vi "Link Control References.vi"(8 "error in (no error)":errorcluster, 10 "Control References":T1[](array[typedef]), 11 "Main in":refnum<class "Main.lvclass">) -> (0 "error out":errorcluster, 3 "Main out":refnum<class "Main.lvclass">)   [LabVIEW 2023, in "Main.lvlib" / "Main.lvclass"]
doc: "<b> Link Control References </b>\n<b> Engine Level </b>\nThis is the base abstraction layer. The purpose of this method is to link the control references to the class private data."
uses:
  Library/Main.lvclass
  builds/Framework/Engine.lvlibp/Engine/Custom Controls/Control Reference.ctl
  Library/Main.lvclass/Main.ctl
  builds/Framework/Engine.lvlibp/Engine/Accessors/Read Version.vi
  builds/Framework/Panel Manager.lvlibp/Panel/Panel/Subpanel/Subpanel.vi
  builds/Framework/Panel Manager.lvlibp/Panel/Panel.lvlib
  builds/Framework/Panel Manager.lvlibp/Panel/Panel/Subpanel/Subpanel.lvclass
  builds/Framework/Engine.lvlibp/Engine/Library/Engine.lvclass
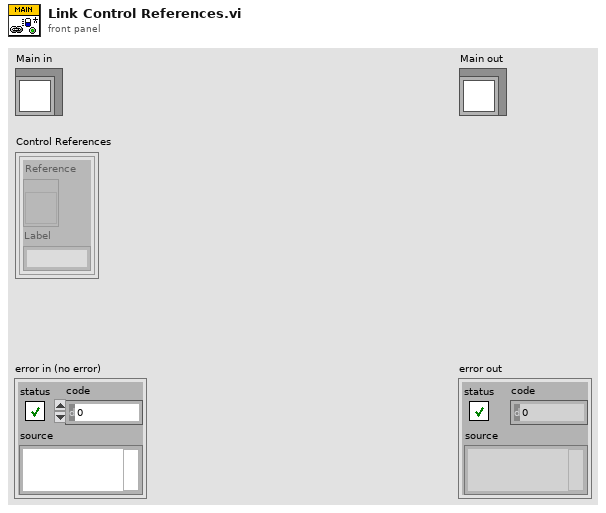
[diagram p1: front panel]
types:
  T1 = typedef "Engine.lvlibp/Engine.lvclass/Control Reference.ctl" = cluster{"Reference":refnum<vi>, "Label":string}
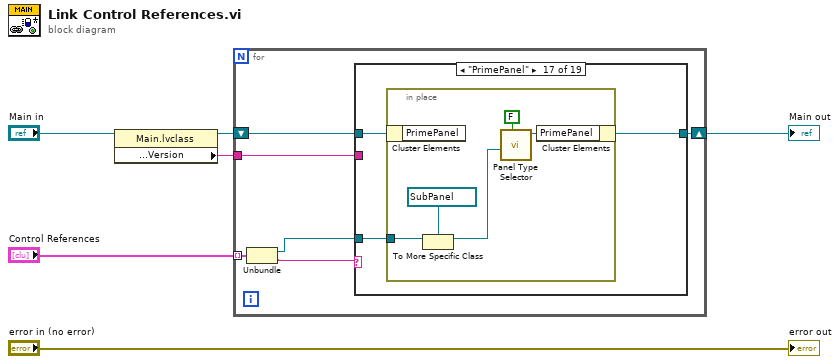
[diagram p0: block diagram]
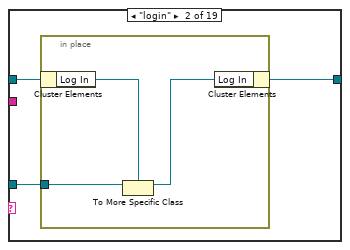
[diagram p3: hidden frame]
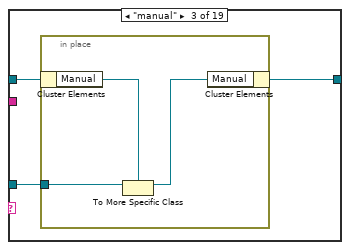
[diagram p4: hidden frame]
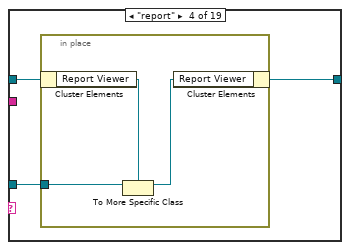
[diagram p5: hidden frame]
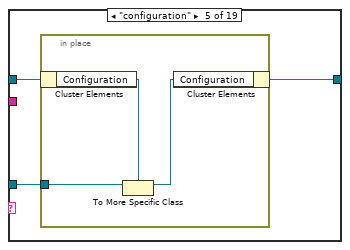
[diagram p6: hidden frame]
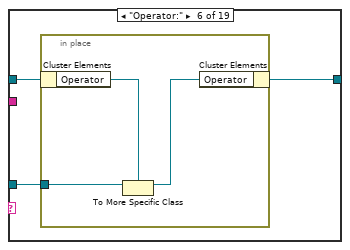
[diagram p7: hidden frame]
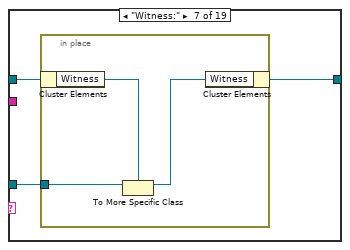
[diagram p8: hidden frame]
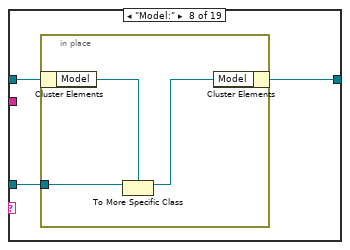
[diagram p9: hidden frame]
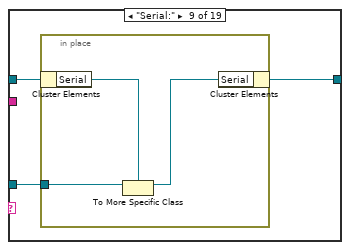
[diagram p10: hidden frame]
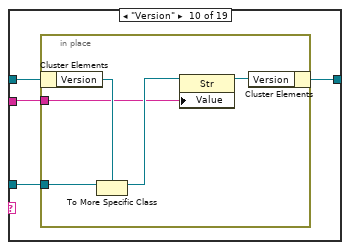
[diagram p11: hidden frame]
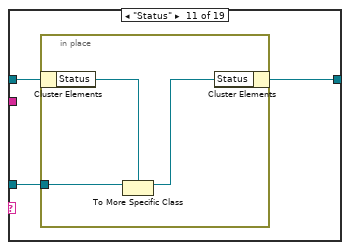
[diagram p12: hidden frame]
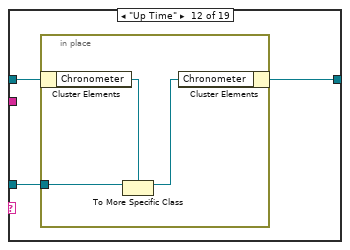
[diagram p13: hidden frame]
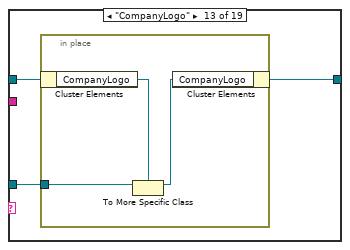
[diagram p14: hidden frame]
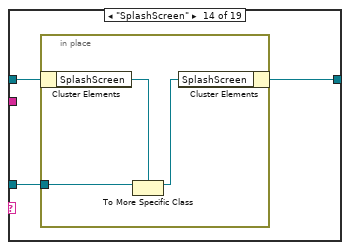
[diagram p15: hidden frame]
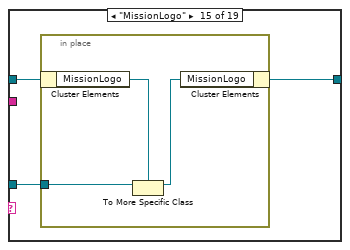
[diagram p16: hidden frame]
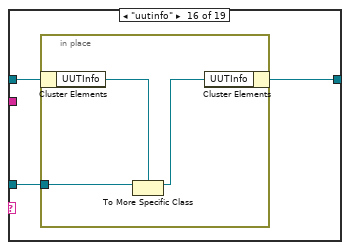
[diagram p17: hidden frame]
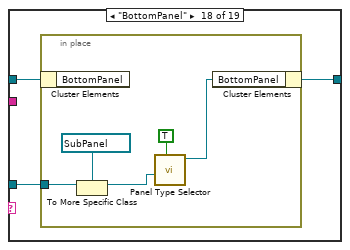
[diagram p18: hidden frame]
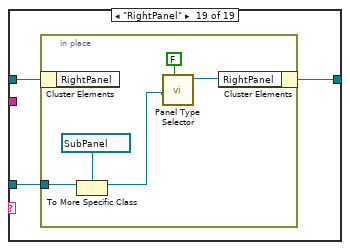
[diagram p19: hidden frame]
diagram:
  n1 = property class="Main.lvclass"(reference="Main in") -> (reference out=w2:refnum<class "Main.lvclass">, "Accessors:Configuration:Version"=w1:string)  [unwired: 1 in, 1 out]
  n2 = for {
    shift-right: [w11] -> w3
    shift-left: w2 -> [w12]
    tunnel: w1 -> [w10]
    tunnel: "Control References" -> [w9] mode=indexing
    n3 = Unbundle(w9) -> ("Reference"=w7:refnum<vi>, "Label"=w8:string)
    n4 = case shown="\"PrimePanel\"" w8 {
      tunnel: w7 -> [_ w14 w20 w26 w32 w38 w44 w50 w56 w63 w71 w77 w83 w89 w95 w101 w107 w115 w123]
      tunnel: w12 -> [w13 w16 w22 w28 w34 w40 w46 w52 w58 w65 w73 w79 w85 w91 w97 w103 w109 w117 w125]
      tunnel: [w13 w15 w21 w27 w33 w39 w45 w51 w57 w64 w72 w78 w84 w90 w96 w102 w108 w116 w124] -> w11
      tunnel: w10 -> [_ _ _ _ _ _ _ _ _ w62 _ _ _ _ _ _ _ _ _]
      frame "False", Default {
      }
      frame "login" {
        n5 = in-place {
          in-place-border: w14 -> [w18]
          n6 = in-place-cluster #1(w16) -> ("Log In"=w19:refnum<vi>)
          n7 = To More Specific Class(target class=w19, reference=w18) -> (specific class reference=w17:refnum<vi>)  [unwired: 1 in, 1 out]
          n8 = in-place-cluster #1("Log In"=w17) -> (w15:refnum<class "Main.lvclass">)
        }
      }
      frame "manual" {
        n9 = in-place {
          in-place-border: w20 -> [w24]
          n10 = in-place-cluster #2(w22) -> ("Manual"=w25:refnum<vi>)
          n11 = To More Specific Class(target class=w25, reference=w24) -> (specific class reference=w23:refnum<vi>)  [unwired: 1 in, 1 out]
          n12 = in-place-cluster #2("Manual"=w23) -> (w21:refnum<class "Main.lvclass">)
        }
      }
      frame "report" {
        n13 = in-place {
          in-place-border: w26 -> [w30]
          n14 = in-place-cluster #3(w28) -> ("Report Viewer"=w31:refnum<vi>)
          n15 = To More Specific Class(target class=w31, reference=w30) -> (specific class reference=w29:refnum<vi>)  [unwired: 1 in, 1 out]
          n16 = in-place-cluster #3("Report Viewer"=w29) -> (w27:refnum<class "Main.lvclass">)
        }
      }
      frame "configuration" {
        n17 = in-place {
          in-place-border: w32 -> [w36]
          n18 = in-place-cluster #4(w34) -> ("Configuration"=w37:refnum<vi>)
          n19 = To More Specific Class(target class=w37, reference=w36) -> (specific class reference=w35:refnum<vi>)  [unwired: 1 in, 1 out]
          n20 = in-place-cluster #4("Configuration"=w35) -> (w33:refnum<class "Main.lvclass">)
        }
      }
      frame "Operator:" {
        n21 = in-place {
          in-place-border: w38 -> [w42]
          n22 = in-place-cluster #5(w40) -> ("Operator"=w43:refnum<vi>)
          n23 = To More Specific Class(target class=w43, reference=w42) -> (specific class reference=w41:refnum<vi>)  [unwired: 1 in, 1 out]
          n24 = in-place-cluster #5("Operator"=w41) -> (w39:refnum<class "Main.lvclass">)
        }
      }
      frame "Witness:" {
        n25 = in-place {
          in-place-border: w44 -> [w48]
          n26 = in-place-cluster #6(w46) -> ("Witness"=w49:refnum<vi>)
          n27 = To More Specific Class(target class=w49, reference=w48) -> (specific class reference=w47:refnum<vi>)  [unwired: 1 in, 1 out]
          n28 = in-place-cluster #6("Witness"=w47) -> (w45:refnum<class "Main.lvclass">)
        }
      }
      frame "Model:" {
        n29 = in-place {
          in-place-border: w50 -> [w54]
          n30 = in-place-cluster #7(w52) -> ("Model"=w55:refnum<vi>)
          n31 = To More Specific Class(target class=w55, reference=w54) -> (specific class reference=w53:refnum<vi>)  [unwired: 1 in, 1 out]
          n32 = in-place-cluster #7("Model"=w53) -> (w51:refnum<class "Main.lvclass">)
        }
      }
      frame "Serial:" {
        n33 = in-place {
          in-place-border: w56 -> [w60]
          n34 = in-place-cluster #8(w58) -> ("Serial"=w61:refnum<vi>)
          n35 = To More Specific Class(target class=w61, reference=w60) -> (specific class reference=w59:refnum<vi>)  [unwired: 1 in, 1 out]
          n36 = in-place-cluster #8("Serial"=w59) -> (w57:refnum<class "Main.lvclass">)
        }
      }
      frame "Version" {
        n37 = in-place {
          in-place-border: w63 -> [w69]
          in-place-border: w62 -> [w66]
          n38 = in-place-cluster #9(w65) -> ("Version"=w70:refnum<vi>)
          n39 = To More Specific Class(target class=w70, reference=w69) -> (specific class reference=w68:refnum<vi>)  [unwired: 1 in, 1 out]
          n40 = property class="Str"(reference=w68, "Value"=w66) -> (reference out=w67:refnum<vi>)  [unwired: 1 in, 1 out]
          n41 = in-place-cluster #9("Version"=w67) -> (w64:refnum<class "Main.lvclass">)
        }
      }
      frame "Status" {
        n42 = in-place {
          in-place-border: w71 -> [w75]
          n43 = in-place-cluster #10(w73) -> ("Status"=w76:refnum<vi>)
          n44 = To More Specific Class(target class=w76, reference=w75) -> (specific class reference=w74:refnum<vi>)  [unwired: 1 in, 1 out]
          n45 = in-place-cluster #10("Status"=w74) -> (w72:refnum<class "Main.lvclass">)
        }
      }
      frame "Up Time" {
        n46 = in-place {
          in-place-border: w77 -> [w81]
          n47 = in-place-cluster #11(w79) -> ("Chronometer"=w82:refnum<vi>)
          n48 = To More Specific Class(target class=w82, reference=w81) -> (specific class reference=w80:refnum<vi>)  [unwired: 1 in, 1 out]
          n49 = in-place-cluster #11("Chronometer"=w80) -> (w78:refnum<class "Main.lvclass">)
        }
      }
      frame "CompanyLogo" {
        n50 = in-place {
          in-place-border: w83 -> [w87]
          n51 = in-place-cluster #12(w85) -> ("CompanyLogo"=w88:refnum<vi>)
          n52 = To More Specific Class(target class=w88, reference=w87) -> (specific class reference=w86:refnum<vi>)  [unwired: 1 in, 1 out]
          n53 = in-place-cluster #12("CompanyLogo"=w86) -> (w84:refnum<class "Main.lvclass">)
        }
      }
      frame "SplashScreen" {
        n54 = in-place {
          in-place-border: w89 -> [w93]
          n55 = in-place-cluster #13(w91) -> ("SplashScreen"=w94:refnum<vi>)
          n56 = To More Specific Class(target class=w94, reference=w93) -> (specific class reference=w92:refnum<vi>)  [unwired: 1 in, 1 out]
          n57 = in-place-cluster #13("SplashScreen"=w92) -> (w90:refnum<class "Main.lvclass">)
        }
      }
      frame "MissionLogo" {
        n58 = in-place {
          in-place-border: w95 -> [w99]
          n59 = in-place-cluster #14(w97) -> ("MissionLogo"=w100:refnum<vi>)
          n60 = To More Specific Class(target class=w100, reference=w99) -> (specific class reference=w98:refnum<vi>)  [unwired: 1 in, 1 out]
          n61 = in-place-cluster #14("MissionLogo"=w98) -> (w96:refnum<class "Main.lvclass">)
        }
      }
      frame "uutinfo" {
        n62 = in-place {
          in-place-border: w101 -> [w105]
          n63 = in-place-cluster #15(w103) -> ("UUTInfo"=w106:refnum<vi>)
          n64 = To More Specific Class(target class=w106, reference=w105) -> (specific class reference=w104:refnum<vi>)  [unwired: 1 in, 1 out]
          n65 = in-place-cluster #15("UUTInfo"=w104) -> (w102:refnum<class "Main.lvclass">)
        }
      }
      frame "PrimePanel" {
        n66 = in-place {
          in-place-border: w107 -> [w114]
          n67 = in-place-cluster #16(w109) -> ()  [unwired: 1 out]
          n68 = To More Specific Class(target class=refnum<vi> refnum ("Sub Panel"), reference=w114) -> (specific class reference=w110:refnum<vi>)  [unwired: 1 in, 1 out]
          n69 = call-poly "Panel Type Selector.vi"("Autoshow? (T)"=FALSE, "Sub Panel"=w110) -> ("Subpanel Out"=w112:refnum<class "Subpanel.lvclass">)  [unwired: 8 in, 1 out]
          n70 = in-place-cluster #16("PrimePanel"=w112) -> (w108:refnum<class "Main.lvclass">)
        }
      }
      frame "BottomPanel" {
        n71 = in-place {
          in-place-border: w115 -> [w122]
          n72 = in-place-cluster #17(w117) -> ()  [unwired: 1 out]
          n73 = To More Specific Class(target class=refnum<vi> refnum ("Sub Panel"), reference=w122) -> (specific class reference=w119:refnum<vi>)  [unwired: 1 in, 1 out]
          n74 = call-poly "Panel Type Selector.vi"("Autoshow? (T)"=TRUE, "Sub Panel"=w119) -> ("Subpanel Out"=w118:refnum<class "Subpanel.lvclass">)  [unwired: 8 in, 1 out]
          n75 = in-place-cluster #17("BottomPanel"=w118) -> (w116:refnum<class "Main.lvclass">)
        }
      }
      frame "RightPanel" {
        n76 = in-place {
          in-place-border: w123 -> [w130]
          n77 = in-place-cluster #18(w125) -> ()  [unwired: 1 out]
          n78 = To More Specific Class(target class=refnum<vi> refnum ("Sub Panel"), reference=w130) -> (specific class reference=w126:refnum<vi>)  [unwired: 1 in, 1 out]
          n79 = call-poly "Panel Type Selector.vi"("Autoshow? (T)"=FALSE, "Sub Panel"=w126) -> ("Subpanel Out"=w128:refnum<class "Subpanel.lvclass">)  [unwired: 8 in, 1 out]
          n80 = in-place-cluster #18("RightPanel"=w128) -> (w124:refnum<class "Main.lvclass">)
        }
      }
    }
  }
  "Main out" <- w3
  "error out" <- "error in (no error)"
